vi "Auto Detect Arduino.vi"(0 "Visa Resource":refnum<visa-resource-name>, 11 "error in (no error)":errorcluster) -> (4 "VISA resource":refnum<visa-resource-name>, 15 "error out":errorcluster)   [LabVIEW 2011, in "LabVIEW Interface for Arduino.lvlib"]
doc: "This VI finds the VISA Resource Names of all COM ports on the host machine. It first finds the VISA Resource Names of all serial ports and then filters through these to find which of those are COM ports."
uses:
  LabVIEW Interface for Arduino.lvlib
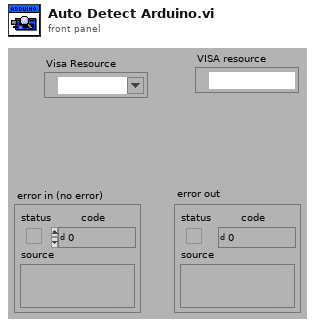
[diagram p1: front panel]
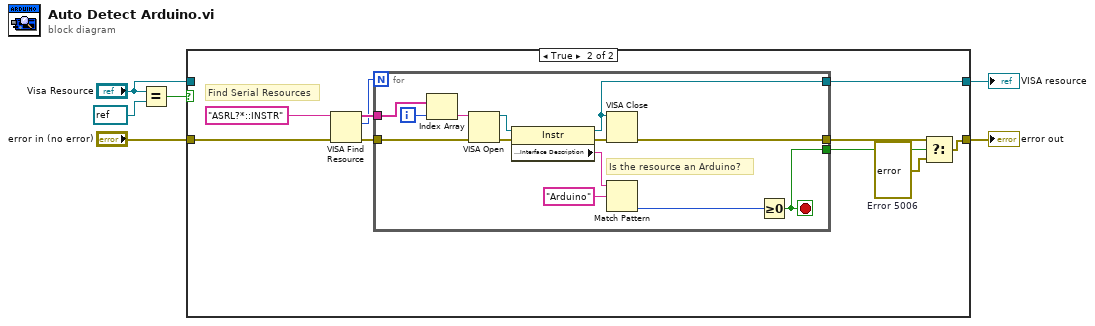
[diagram p0: block diagram]
diagram:
  n1 = Equal?(x="Visa Resource", y=refnum<visa-resource-name> refnum ("VISA resource")) -> (x = y?=w6:bool)
  n2 = case shown="True" w6 {
    tunnel: "error in (no error)" -> [w7 w11]
    tunnel: [w7 w10] -> w3
    tunnel: [w8 w9] -> w2
    tunnel: "Visa Resource" -> [w8 _]
    frame False {
    }
    frame True {
      w18 = errorcluster {"status"=TRUE, "code"=5005, "source"="Unable to find Arduino.  Please make sure the Arduino is connected to your system and that the Arduino drivers are installed."}  # Error 5006
      # "Find Serial Resources"
      n3 = VISA Find Resource(8:w11, 11:"ASRL?*::INSTR" ("expression (\"\")")) -> (0:w15:errorcluster, 2:w13:u32, 3:w14:string[])  [unwired: 1 in]
      n4 = for {
        N: w13 -> [_]
        tunnel: w14 -> [w29]
        tunnel: w15 -> [w22]
        tunnel: [w21] -> w17
        tunnel: [w20] -> w9
        tunnel: [w19] -> w16
        i -> [w25]
        stop <- w19 stop-if-true
        # "Is the resource an Arduino?"
        n5 = Index Array(array=w29, index=w25) -> (element=w23:string)
        n6 = VISA Open(error in (no error)=w22, VISA resource name=w23) -> (VISA resource name=w24:refnum<visa-resource-name>, error out=w31:errorcluster)  [unwired: 3 in]
        n7 = property class="Instr"(reference=w24, error in=w31) -> (reference out=w20:refnum<visa-resource-name>, error out=w30:errorcluster, "Interface Information:Interface Description"=w28:string)
        n8 = VISA Close(VISA resource name=w20, error in (no error)=w30) -> (error out=w21:errorcluster)
        n9 = Match Pattern(string=w28, regular expression="Arduino") -> (offset past match=w26:i32)  [unwired: 1 in, 3 out]
        n10 = Greater Or Equal To 0?(x=w26) -> (x >= 0?=w19:bool)
      }
      n11 = Select(t=w17, s=w16, f=w18) -> (s? t:f=w10:errorcluster)
    }
  }
  "error out" <- w3
  "VISA resource" <- w2
